vi "LoggingHeaders.vi"(8 "error in":errorcluster, 10 "Date and Time":string, 11 "refnum in":refnum<file>) -> (0 "error out":errorcluster, 3 "refnum out":refnum<file>)   [LabVIEW 2017]
uses:
  LogOperation.ctl
  <vilib>/Rock Robotics/Network Tables/NT Read Number.vi
  <vilib>/Rock Robotics/Network Tables/NT Read String.vi
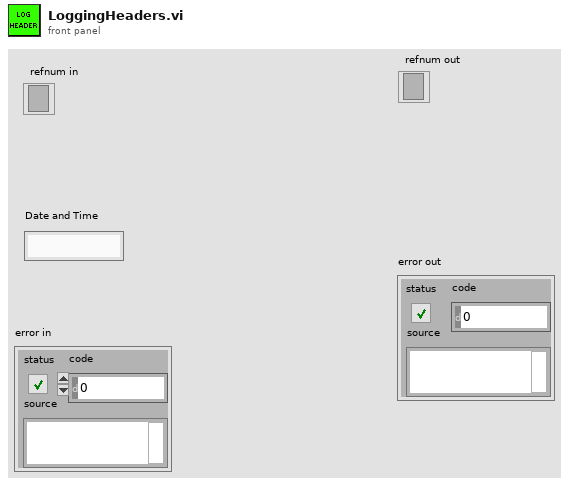
[diagram p1: front panel]
types:
  T1 = typedef "LogOperation.ctl" = enum16{"Set", "Get All", "Init"}
  T2 = typedef "NetComm_MatchType.ctl" = enum32{"None", "Practice", "Qualification", "Elimination"}
  T3 = typedef "WPI_DriverStationPositionInfo.ctl" = enum16{"1", "2", "3"}
  T4 = typedef "WPI_DriverStationAllianceInfo.ctl" = enum16{"Red", "Blue", "Invalid"}
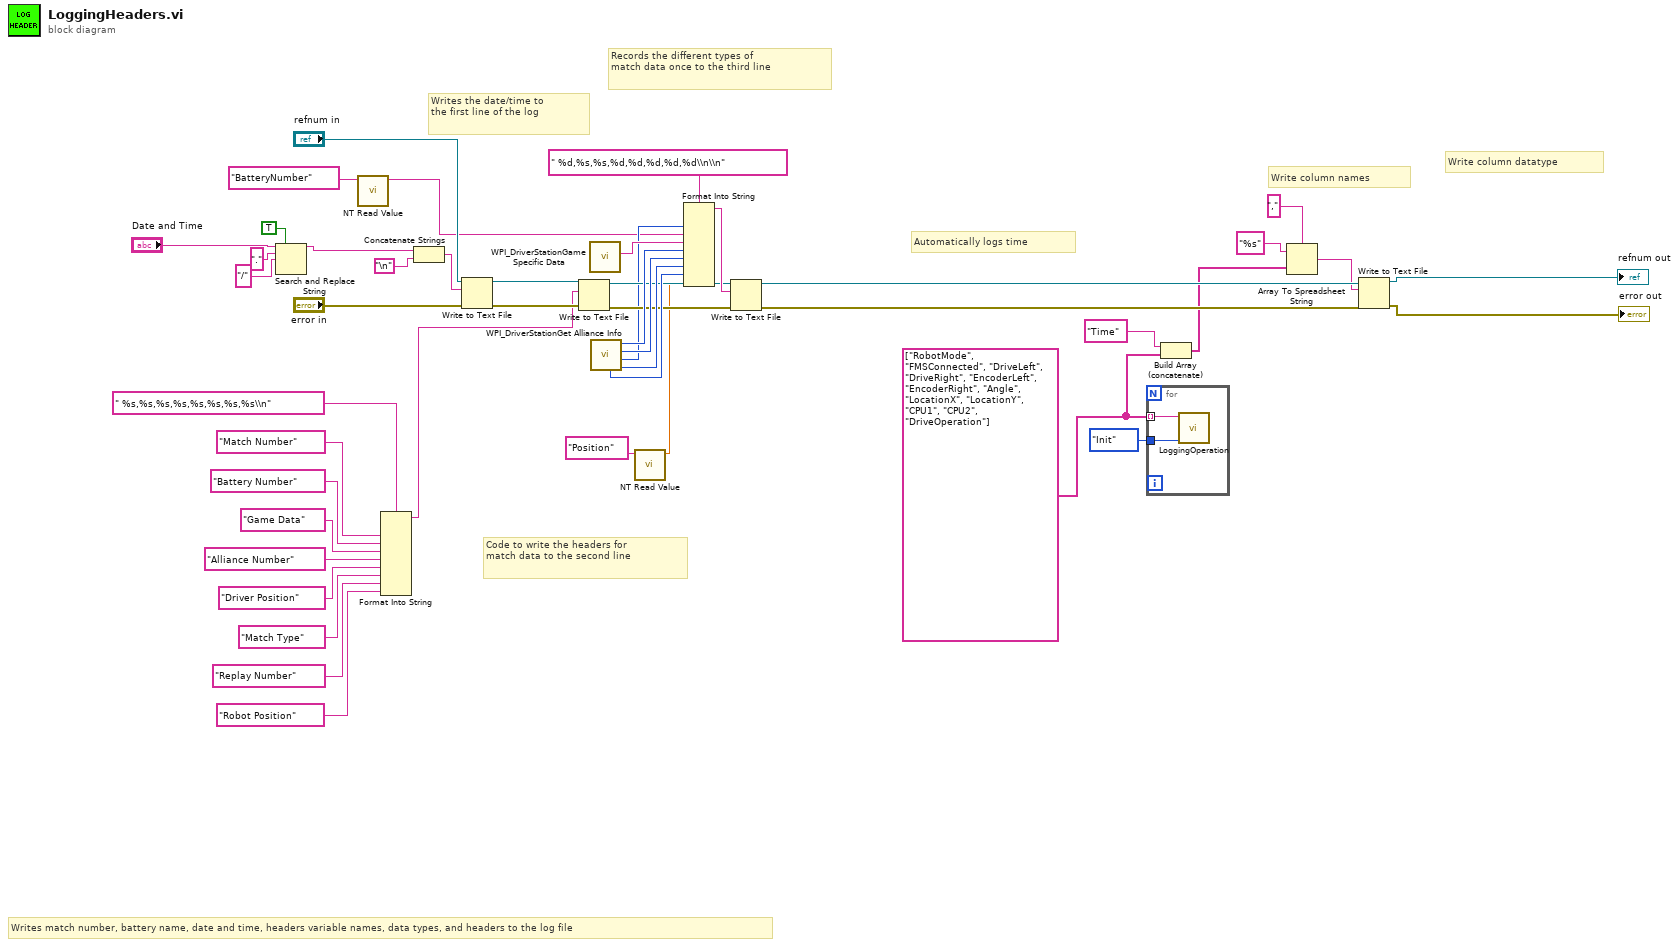
[diagram p0: block diagram]
diagram:
  w2 = string[] ["RobotMode", "FMSConnected", "DriveLeft", "DriveRight", "EncoderLeft", "EncoderRight", "Angle", "LocationX", "LocationY", "CPU1", "CPU2", "DriveOperation"] ("Column Names")
  # "Automatically logs time"
  # "Write column datatype"
  # "Write column names"
  # "Records the different types of \nmatch data once to the third line"
  # "Code to write the headers for \nmatch data to the second line"
  # "Writes the date/time to\nthe first line of the log"
  # "Writes match number, battery name, date and time, headers variable names, data types, and headers to the log file"
  n1 = Search and Replace String(replace all?=TRUE ("replace all? (F)"), input string="Date and Time", search string=".", replace string="/" ("search string")) -> (result string=w12:string)  [unwired: 4 in, 3 out]
  n2 = call-poly <vilib>:"NT Read Value.vi"("Name"="BatteryNumber") -> ("String"=w6:string)  [unwired: 9 in, 1 out]
  n3 = Format Into String(format string=" %s,%s,%s,%s,%s,%s,%s,%s\\n", "Match Number" ("input 2"), "Battery Number" ("input 2"), "Game Data" ("input 2"), "Alliance Number" ("input 2"), "Driver Position" ("input 2"), "Match Type" ("input 2"), "Replay Number" ("input 2"), "Robot Position" ("input 2")) -> (resulting string=w17:string)  [unwired: 2 in, 1 out]
  n4 = Concatenate Strings(w12, "\n") -> (w45:string)
  n5 = Write to Text File(file (use dialog)="refnum in", text=w45, error in="error in") -> (refnum out=w29:refnum<file>, error out=w28:errorcluster)  [unwired: 1 in, 1 out]
  n6 = Write to Text File(file (use dialog)=w29, text=w17, error in=w28) -> (refnum out=w26:refnum<file>, error out=w27:errorcluster)  [unwired: 1 in, 1 out]
  n7 = call <vilib>:"WPI_DriverStationGame Specific Data.vi"() -> ("Game Specific Data"=w34:string)  [unwired: 11 in]
  n8 = call <vilib>:"WPI_DriverStationGet Alliance Info.vi"() -> ("Match Type"=w31:T2, "Match Number"=w8:u16, "Position"=w32:T3, "Alliance"=w33:T4, "Replay Number"=w30:u16)  [unwired: 6 in, 1 out]
  n9 = call-poly <vilib>:"NT Read Value.vi"("Name"="Position") -> ("Numeric"=w9:dbl)  [unwired: 9 in, 1 out]
  n10 = Format Into String(format string=" %d,%s,%s,%d,%d,%d,%d,%d\\n\\n", w8, w6, w34, w33, w32, w31, w30, w9) -> (resulting string=w42:string)  [unwired: 2 in, 1 out]
  n11 = Write to Text File(file (use dialog)=w26, text=w42, error in=w27) -> (refnum out=w40:refnum<file>, error out=w39:errorcluster)  [unwired: 1 in, 1 out]
  n12 = for {
    tunnel: w2 -> [w48] mode=indexing
    tunnel: LogOperation."Init" ("Operation") -> [w47]
    n13 = call "LoggingOperation.vi"("Operation"=w47, "Name"=w48) -> ()  [unwired: 9 in, 1 out]
  }
  n14 = Build Array (concatenate)("Time" ("Column Name"), w2) -> (w1:string[])
  n15 = Array To Spreadsheet String(delimiter (Tab)=",", array=w1, 3:"%s" ("format string")) -> (spreadsheet string=w36:string)
  n16 = Write to Text File(file (use dialog)=w40, text=w36, error in=w39) -> (refnum out=→"refnum out":refnum<file>, error out=→"error out":errorcluster)  [unwired: 1 in, 1 out]
